vi "Emballage_BDD_PRINT_continuer_Cmd_sans_melange_des_lots.vi"(8 "error in (no error)":errorcluster caption="entrée d'erreur (pas d'erreur)", 9 "Carton prochain Numéro":i16, 10 "N° carton":u8=1, 11 "Tableau \nlots OUT":string[][](array[string])) -> (0 "error out":errorcluster caption="sortie d'erreur")   [LabVIEW 2020]
uses:
  Modules/FS/60_FS_Controles/60_FS_SetGet.ctl
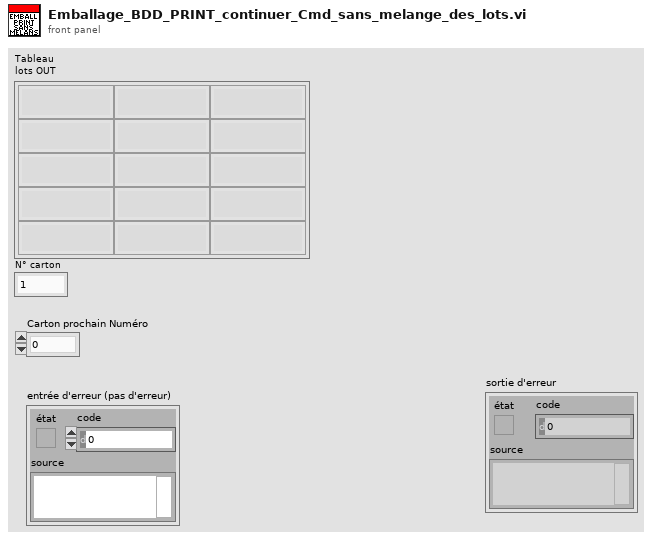
[diagram p1: front panel]
types:
  T1 = enum16{"n° produit", "date", "opérateur", "n° cmde", "n° carton", "qtté cmdée ou retour client"}
  T2 = typedef "60_FS_SetGet.ctl" = enum16{"set", "get"}
  T3 = typedef "DATA commande.ctl" = cluster{"n°article FAS":string, "n° cmde FAS":string, "quantité cmde":string, "ID LIG cmde":string, "n° cmde client":string, "nom client":string, "n° article client":string, "indice revision client":string, "société de facturation":string, "langue a utiliser":string}
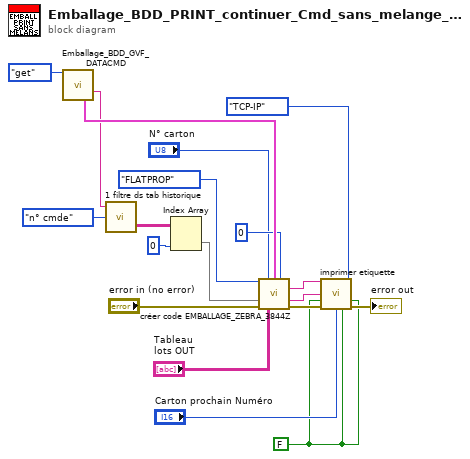
[diagram p0: block diagram]
diagram:
  w8 = FALSE ("sélecteur")
  n1 = call "Emballage_BDD_GVF_DATACMD.vi"("SetGet"=60_FS_SetGet."get") -> ("No commande FAS OUT"=w4:string, "DATA cmde OUT"=w18:T3)  [unwired: 7 in, 6 out]
  n2 = call "1 filtre ds tab historique.vi"("Filtre"=T1."n° cmde", "valeur recherchée"=w4) -> ("Tab historique filtré par ordre croissant carton"=w2:string[][])  [unwired: 1 in, 1 out]
  n3 = Index Array(array=w2, index (col)=0) -> (element=w1:string[])  [unwired: 1 in]
  n4 = call "créer code EMBALLAGE_ZEBRA_3844Z.vi"("DIVISION"=enum16{"FLATPROP", "MEDIC"}."FLATPROP", "N° carton"="N° carton", "DATA cmde"=w18, "Nb total cartons"=0, "Tableau n° valves"=w1, "error in (no error)"="error in (no error)", "Tableau \nlots OUT"="Tableau \nlots OUT") -> ("chaine  à écrire"=w15:string, "n°article FAS"=w14:string, "error out"=w13:errorcluster)  [unwired: 5 in, 1 out]
  n5 = call "imprimer etiquette.vi"("chaine à écrire"=w15, "Type de liaison"=enum16{"RS232", "USB", "TCP-IP", "Aucune"}."TCP-IP", "n°article FAS"=w14, "sélecteur"=w8, "Cde_Interne"=w8, "error in"=w13, "Carton Numéro"="Carton prochain Numéro", "fin de série ?"=w8) -> ("error out"=→"error out":errorcluster)  [unwired: 7 in]
